vi "Menu.vi"(7 "Name (\"\" to Use UUID)":string="Menu") -> ()   [LabVIEW 2025]
doc: "Compact code template used to create a CSM module with a user interface. This template includes a user Event Structure for responding to user actions. The functionality of this template is identical to the CSM User Interface(UI) Module Template VI.\n\n\n> [!NOTE] <b>CSM Naming Rules</b>\n>\n> - CSM module name must be unique. Otherwise, CSM enters a `Critical Error` state.\n> - If the input module name is an empty string (\"\"), the system uses a UUID as the module name. Such a module is marked as standalone mode and does not appear in the module list.\n> - Worker Mode Rule: If the input module name ends with `#`, a worker mode node will be instantiated. Multiple worker mode nodes can form a worker mode module.\n> - Chain of Responsibility Mode Rule: If the input module name ends with `$` followed by a number, a chain of responsibility mode node will be instantiated. Multiple chain of responsibility mode nodes can form a chain of responsibility mode module.\n> - System-Level Module Rule: If the input module name starts with `.`, the module is a system-level module. Under default settings, such modules are not listed by the CSM - List Modules VI and are suitable for instantiating modules that run in the background.\n> - Submodule Rule: `.` is also allowed in a module name to separate the module name into multiple parts. CSM does not have strict rules for submodules. The `.` in the module name only marks the logical relationship between different modules. From an execution perspective, they are considered independent modules. The only difference is that you can obtain a list of logical submodules via the CSM - List Submodules VI.\n\n\n-- <b>Controls</b> --\n- <b>Name (\"\" to use UUID)</b>: CSM module name. Refer to <b>CSM Naming Rules</b> for module naming rules."
uses:
  <userlib>/_NEVSTOP/Communicable State Machine(CSM)/AdvanceAPI/CSM - Revert Arguments-Safe String.vi
  <userlib>/_NEVSTOP/Communicable State Machine(CSM)/_Shared/Trim Single-line Text.vi
  <userlib>/_NEVSTOP/Communicable State Machine(CSM)/AdvanceAPI/CSM - Break Down Multiple States String.vi
  <userlib>/_NEVSTOP/Communicable State Machine(CSM)/AdvanceAPI/CSM - Compact Multiple States.vi
  <userlib>/_NEVSTOP/Communicable State Machine(CSM)/AdvanceAPI/CSM - Make String Arguments Safe.vi
  <userlib>/_NEVSTOP/Communicable State Machine(CSM)/AdvanceAPI/CSM - Keywords.vi
  <userlib>/_NEVSTOP/Communicable State Machine(CSM)/Communicable State Machine.lvlib
panel:
  out "State History":string
  in  "Tab Control":enum32{"Play", "Rules"}(tab)
  in  "Rules Button":bool
  out "Records Display":string
  in  "Difficulty":enum32{"Eazy", "Hard", "Insane"}(radio)
  in  "Start Button":bool
  in  "Quit":bool
  out "Rules":string
  in  "Back Button":bool
  out "Simon Rules":string
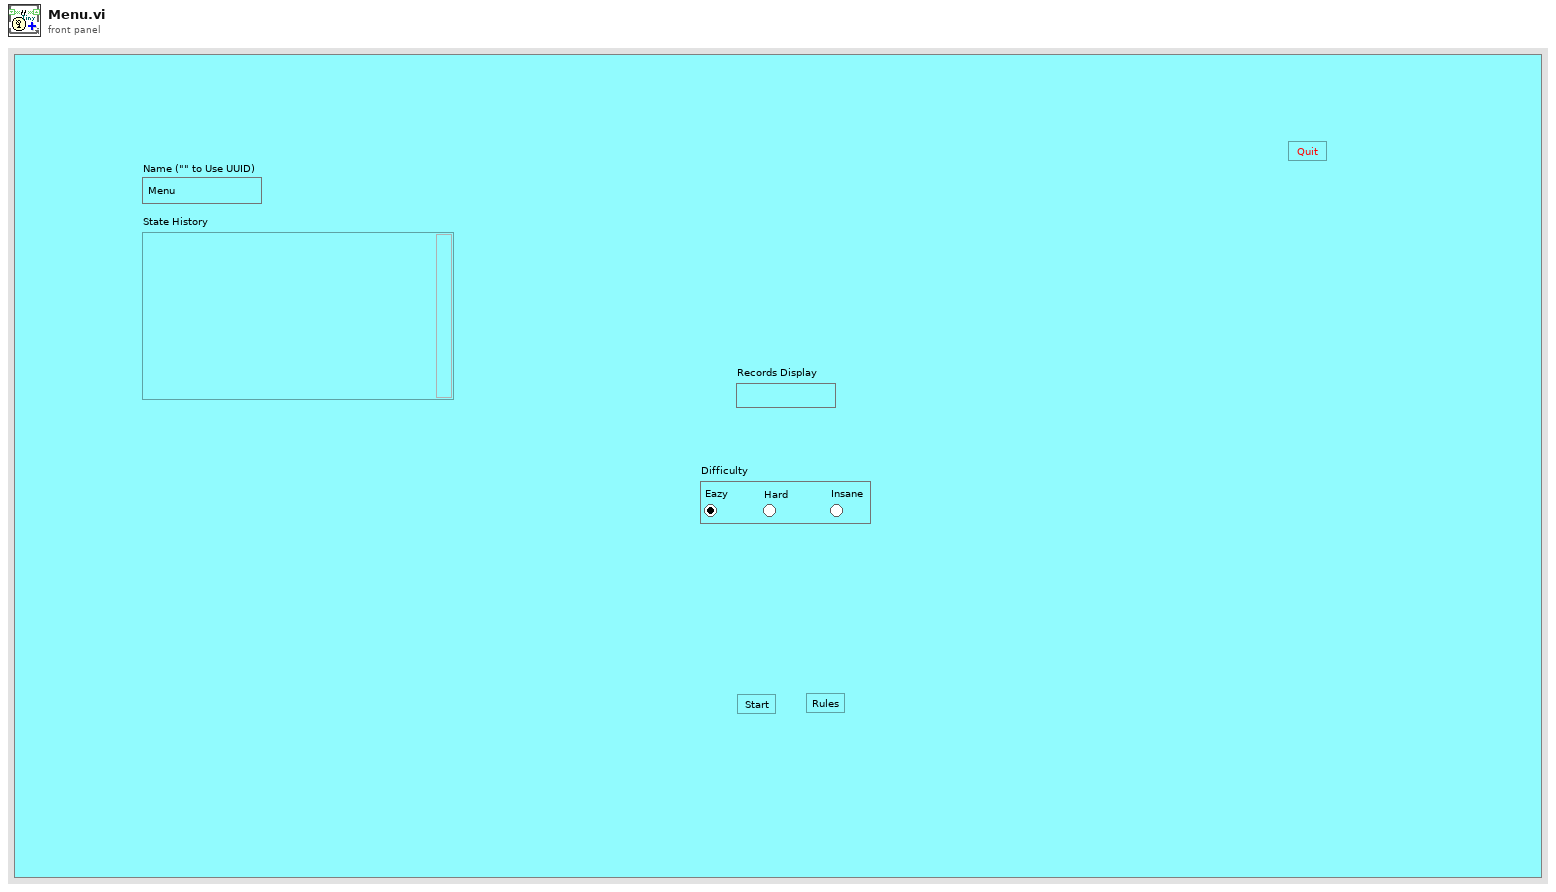
[diagram p1: front panel]
types:
  T1 = enum32{"Invalid", "Standard", "Closed", "Hidden", "Minimized", "Maximized"}
  T2 = enum32{"invalid app kind", "Development System", "Run Time System", "Student Edition", "Embedded LabVIEW", "Evaluation", "Custom"}
  T3 = typedef "Communicable State Machine.lvlib/_CSM_Response Source Message.ctl" = cluster{"‘State":string, "’Arguments":string, "’Error":errorcluster}
  T4 = cluster{"Core":cluster{"Current VI Reference":refnum<vi>, "Close Panel on Exit?":bool}, "Difficulty":i32}
  T5 = cluster{"Current VI Reference":refnum<vi>, "Close Panel on Exit?":bool}
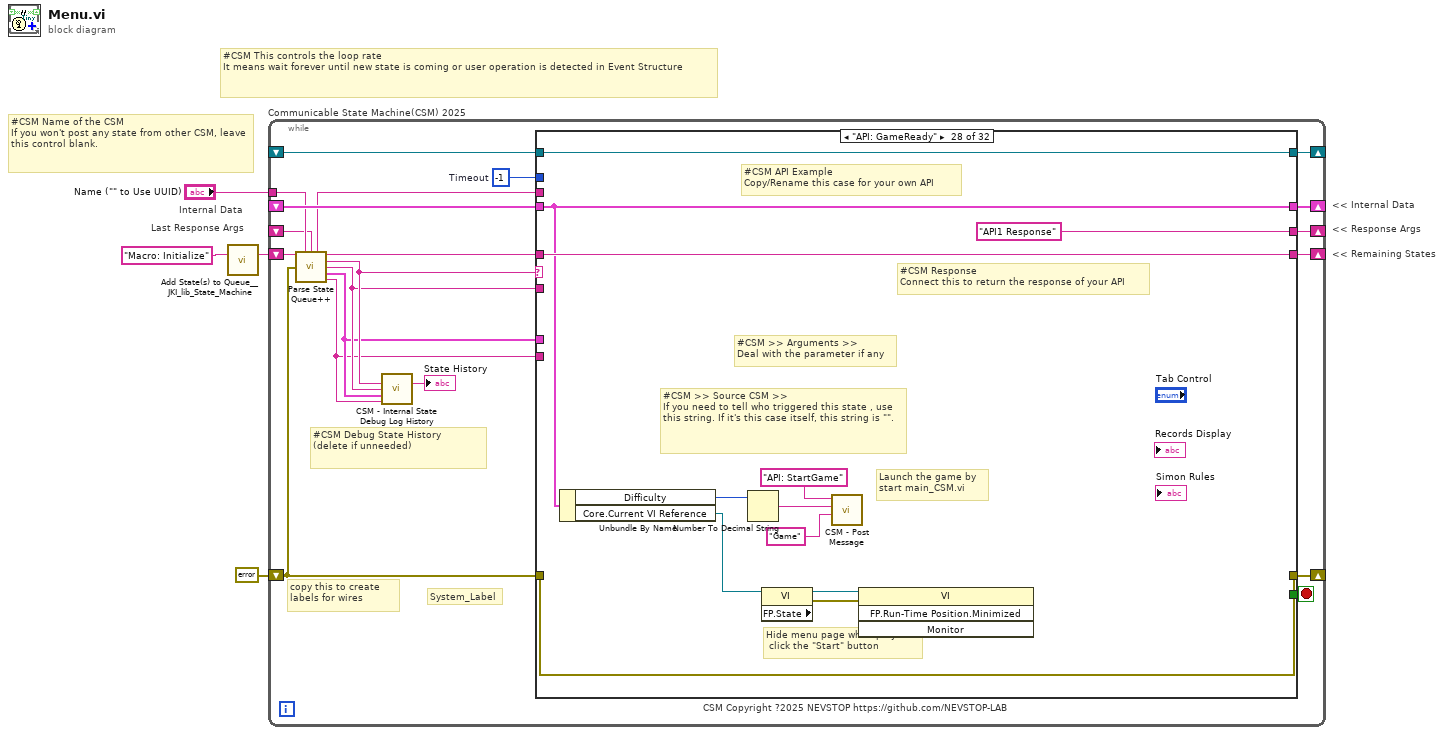
[diagram p0: block diagram]
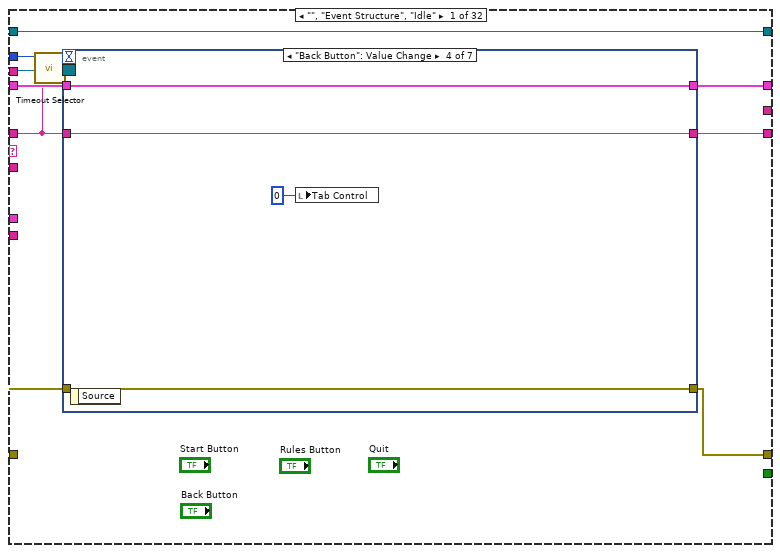
[diagram p2: hidden frame]
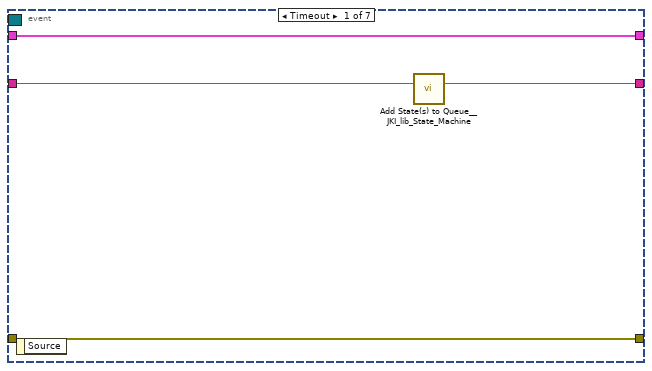
[diagram p3: hidden frame]
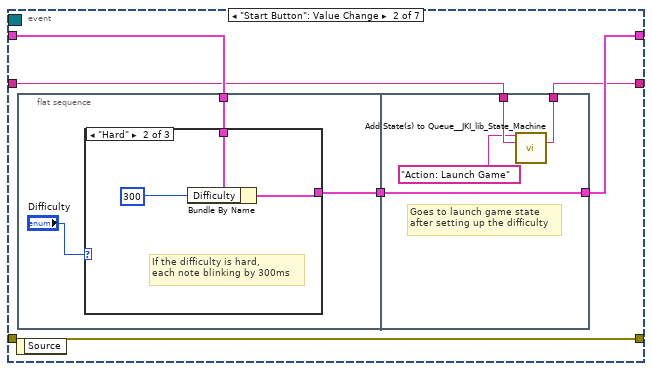
[diagram p4: hidden frame]
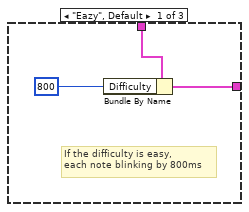
[diagram p5: hidden frame]
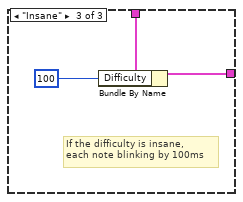
[diagram p6: hidden frame]
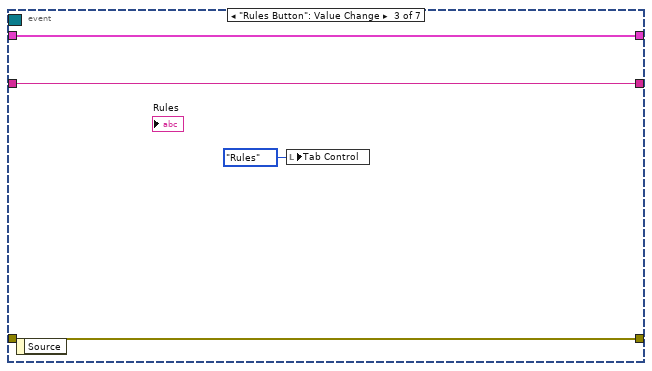
[diagram p7: hidden frame]
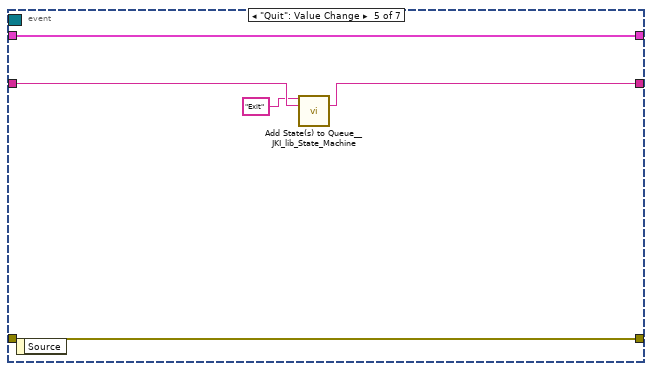
[diagram p8: hidden frame]
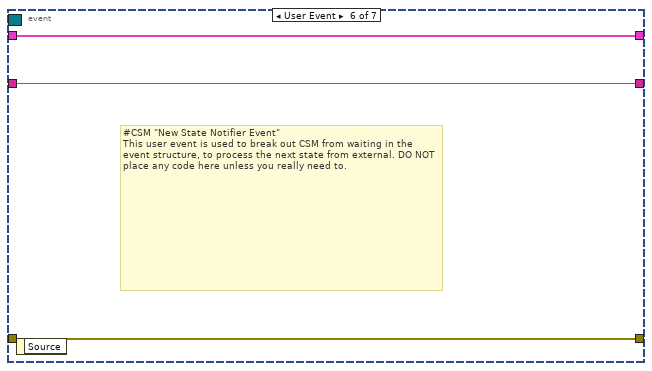
[diagram p9: hidden frame]
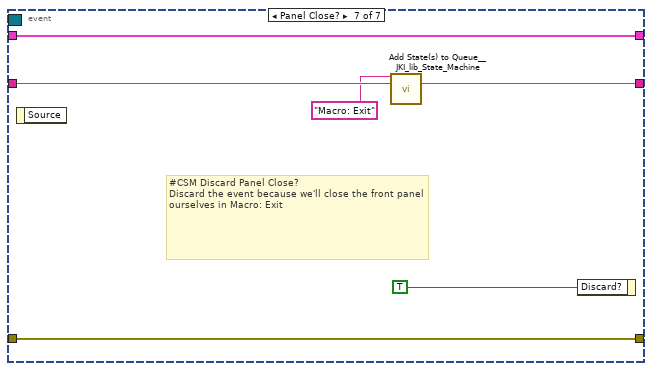
[diagram p10: hidden frame]
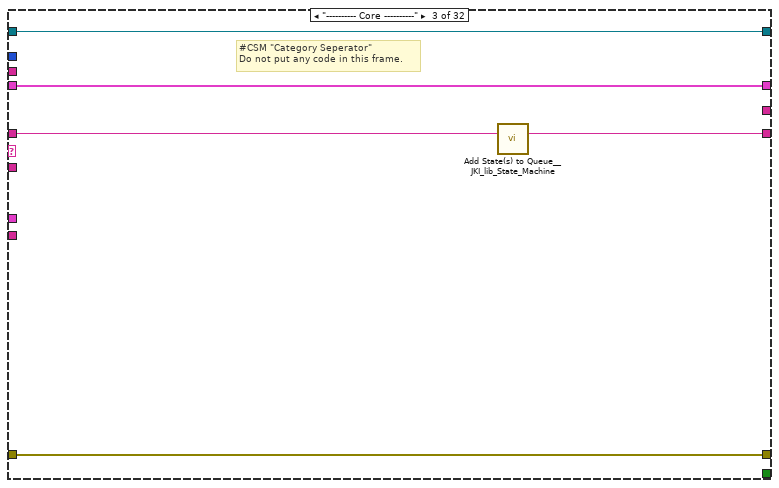
[diagram p12: hidden frame]
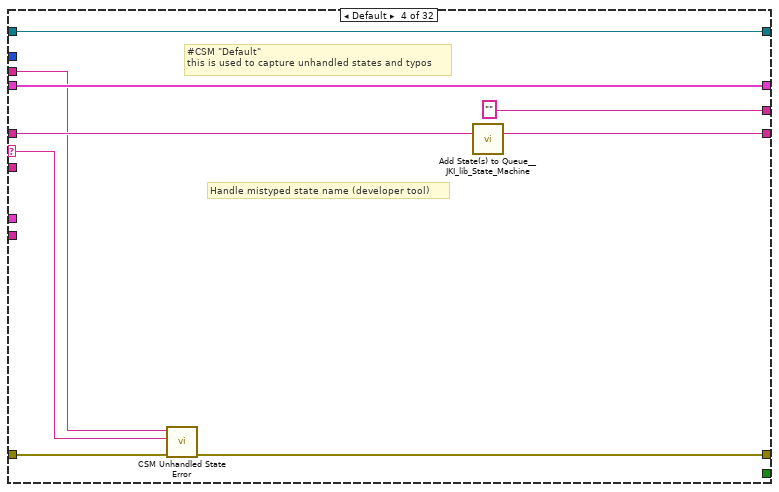
[diagram p13: hidden frame]
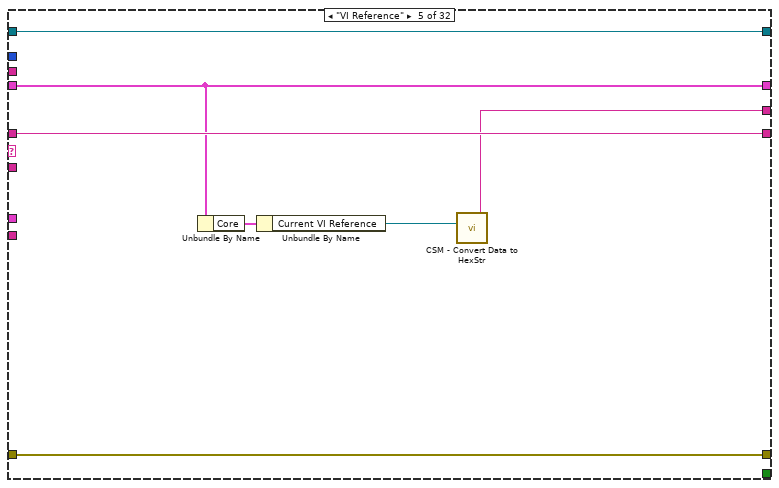
[diagram p14: hidden frame]
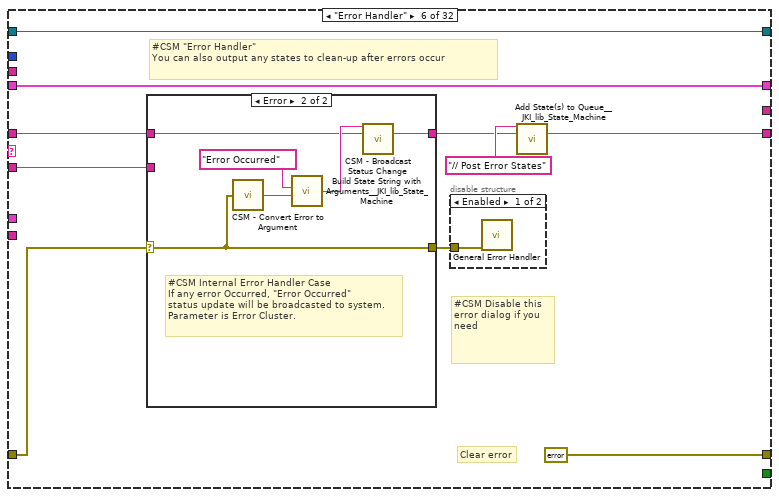
[diagram p15: hidden frame]
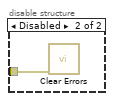
[diagram p16: hidden frame]
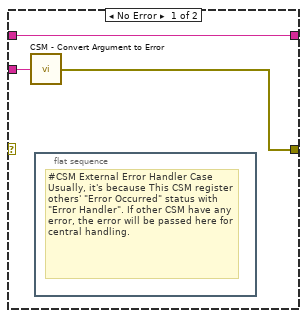
[diagram p17: hidden frame]
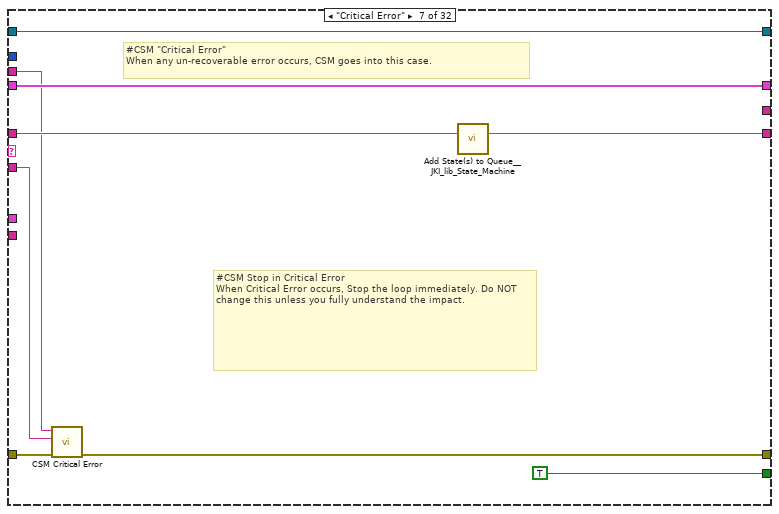
[diagram p18: hidden frame]
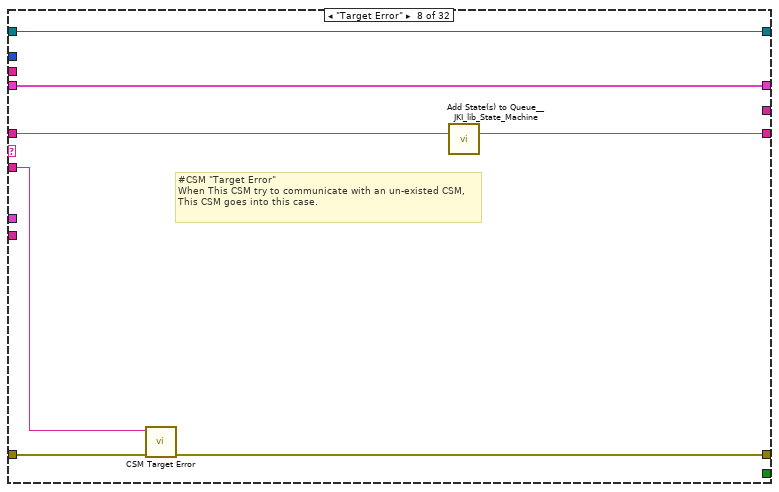
[diagram p19: hidden frame]
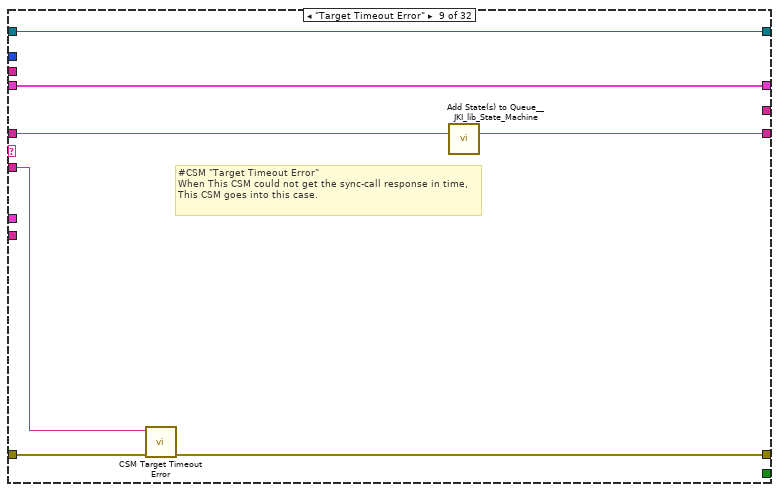
[diagram p20: hidden frame]
diagram:
  # "Last Response Args"
  # "Internal Data"
  # "#CSM Name of the CSM\nIf you won't post any state from other CSM, leave this control blank."
  # "#CSM This controls the loop rate\nIt means wait forever until new state is coming or user operation is detected in Event Structure"
  # "<< Internal Data"
  # "<< Response Args"
  # "<< Remaining States"
  n1 = call <vilib>:"Add State(s) to Queue__JKI_lib_State_Machine.vi"("State(s) in (\"\")"="Macro: Initialize" ("Init State(\"Macro: Initialize\")")) -> ("States Out"=w4:string)  [unwired: 14 in]
  n2 = while "Communicable State Machine(CSM) 2025" {
    shift-right: [w19] -> _
    shift-left: _ -> [w18]
    shift-right: [w22] -> _
    shift-left: errorcluster {"status"=FALSE, "code"=0, "source"=""} ("error out") -> [w16]
    shift-right: [w21] -> _
    shift-left: w4 -> [w23]
    tunnel: "Name (\"\" to Use UUID)" -> [w12]
    shift-right: [w15] -> _
    shift-left: _ -> [w6]
    shift-right: [w14] -> _
    shift-left: _ -> [w13]
    stop <- w20 stop-if-true
    w17 = -1  # Timeout
    # "#CSM Debug State History\n(delete if unneeded)"
    # "copy this to create labels for wires"
    # "System_Label"
    # "CSM Copyright ?2025 NEVSTOP https://github.com/NEVSTOP-LAB"
    n3 = call <userlib>:"Parse State Queue++.vi"("State Queue"=w23, "Name (\"\" to Use UUID)"=w12, "Response Arguments"=w6, "Previous Error"=w16) -> ("Name Used"=w7:string, "Remaining States"=w24:string, "Current State"=w11:string, "Arguments"=w10:string, "Additional Information"=w9:T3, "Source CSM"=w8:string)  [unwired: 6 in]
    n4 = call <userlib>:"CSM - Internal State Debug Log History.vi"("State"=w11, "Arguments (\"\")"=w10, ">> Response Source Message >>"=w9, "Source (\"\")"=w8) -> ("Debug Log"=→"State History":string)  [unwired: 11 in]
    n5 = case shown="\"API: GameReady\"" w11 {
      selector: w11 -> [_ _ _ w93 _ _ _ _ _ _ _ _ _ _ _ _ _ _ _ _ _ _ _ _ _ _ _ _ _ _ _ _]
      tunnel: w24 -> [w25 w84 w90 w98 w105 w111 w134 w140 w147 w156 w169 w184 w190 w195 w202 w209 w214 w221 w225 w231 w236 w243 w259 w329 w335 w347 w350 w362 w368 w376 w388 w393]
      tunnel: w10 -> [_ _ _ _ _ w110 w129 w139 w146 w155 _ _ _ _ _ _ _ _ _ _ _ w238 w253 _ _ _ _ _ w365 _ _ _]
      tunnel: w18 -> [w32 w83 w87 w96 w104 w115 w135 w142 w149 w158 w168 w177 w188 w192 _ w204 w211 w220 w224 w228 w234 w241 w255 w326 w332 w344 w349 w356 w367 w373 w385 w390]
      tunnel: [w31 w85 w88 w91 w106 errorcluster {"status"=FALSE, "code"=0, "source"=""} ("error out") w130 w137 w144 w161 w170 w181 w187 w193 w199 w205 w212 w215 w223 w229 w233 w239 w256 w327 w333 w345 w351 w363 w369 w374 w386 w391] -> w22
      tunnel: w16 -> [w30 w85 w88 w99 w106 w112 w136 w138 w145 _ w170 w181 w187 w193 w199 w206 w212 _ w226 w229 w233 w240 w257 w327 w333 w345 w351 w363 w369 w374 w386 w391]
      tunnel: [w33 w84 w89 w97 w105 w107 w133 w143 w150 w157 w169 w183 w189 w194 w201 w208 w213 w221 w225 w230 w235 w242 w258 w328 w334 w346 w350 w362 w368 w375 w387 w392] -> w21
      tunnel: [_ _ _ _ _ _ TRUE _ _ _ _ _ TRUE _ _ _ _ _ _ _ _ _ _ _ _ _ _ _ _ _ _ _] -> w20
      tunnel: [w29 w83 w87 w96 w104 w115 w135 w142 w149 w159 w168 w182 w188 w192 w200 w204 w211 w220 w224 w228 w234 w241 w255 w326 w332 w344 w349 w356 w367 w373 w385 w390] -> w19
      tunnel: w17 -> [w28 _ _ _ _ _ _ _ _ _ _ _ _ _ _ _ _ _ _ _ _ _ _ _ _ _ _ _ _ _ _ _]
      tunnel: w8 -> [_ _ _ _ _ _ _ _ _ w153 _ _ _ _ _ _ _ _ _ _ _ _ _ _ _ _ _ _ _ _ _ _]
      tunnel: w9 -> [_ _ _ _ _ _ _ _ _ w160 _ _ _ _ _ _ _ _ _ _ _ _ _ _ _ _ _ _ _ _ _ _]
      tunnel: [_ _ _ "" w100 _ _ _ _ _ _ _ _ _ _ _ _ _ _ _ _ _ _ _ _ _ _ "API1 Response" w364 _ _ _] -> w15
      tunnel: [w27 w82 w86 w94 w103 w114 w131 w141 w148 w162 w167 w171 w185 w191 w197 w203 w210 w219 w222 w227 w232 w237 w252 w325 w330 w337 w348 w361 w366 w372 w384 w389] -> w14
      tunnel: w13 -> [w27 w82 w86 w94 w103 w114 w131 w141 w148 w162 w167 w171 w185 w191 w197 w203 w210 _ w222 w227 w232 w237 w252 w325 w330 w337 w348 w361 w366 w372 w384 w389]
      tunnel: w7 -> [_ _ _ w92 _ _ w128 _ _ _ _ _ _ _ _ _ _ w218 _ _ _ _ _ _ _ _ _ _ _ _ _ _]
      frame "", "Event Structure", "Idle" {
        n6 = call <userlib>:"Timeout Selector.vi"("Remaining States"=w25, "Timeout Expected"=w28) -> ("Timeout"=w26:i32)  [unwired: 5 in]
        n7 = event shown="[3] \"Back Button\": Value Change" {
          selector: w27 -> [_ _ _ _ _ _ _]
          dyn-events: _ -> [_ _ _ _ _ _ _]
          timeout: w26 -> [_ _ _ _ _ _ _]
          tunnel: w25 -> [w37 w39 w63 w67 w70 w74 w81]
          tunnel: [w36 w38 w63 w67 w69 w74 w80] -> w33
          tunnel: w32 -> [w34 w42 w61 w65 w71 w75 w78]
          tunnel: [w35 w43 w62 w66 w72 w73 w79] -> w31
          tunnel: w30 -> [w35 w43 w62 w66 w72 w73 w79]
          tunnel: [w34 w41 w61 w65 w71 w75 w78] -> w29
          event Timeout {
            n8 = event-data() -> ()  [unwired: 1 in, 1 out]
            n9 = call <vilib>:"Add State(s) to Queue__JKI_lib_State_Machine.vi"("State(s) in (\"\")"=w37) -> ("States Out"=w36:string)  [unwired: 14 in]
          }
          event "Start Button": Value Change {
            n10 = event-data() -> ()  [unwired: 1 in, 1 out]
            n11 = flat-sequence {
              tunnel: w42 -> [w45]
              tunnel: [w44] -> w40
              tunnel: [w59] -> w41
              tunnel: w40 -> [w59]
              tunnel: w39 -> [w58]
              tunnel: [w57] -> w38
              frame #0 {
                n12 = case shown="\"Hard\"" "Difficulty" {
                  tunnel: w45 -> [w49 w52 w55]
                  tunnel: [w47 w51 w54] -> w44
                  frame "Eazy", Default {
                    # "If the difficulty is easy,\neach note blinking by 800ms"
                    n13 = Bundle By Name(cluster=w49, "Difficulty"=800) -> (w47:T4)
                  }
                  frame "Hard" {
                    # "If the difficulty is hard,\neach note blinking by 300ms"
                    n14 = Bundle By Name(cluster=w52, "Difficulty"=300) -> (w51:T4)
                  }
                  frame "Insane" {
                    # "If the difficulty is insane,\neach note blinking by 100ms"
                    n15 = Bundle By Name(cluster=w55, "Difficulty"=100) -> (w54:T4)
                  }
                }
              }
              frame #1 {
                # "Goes to launch game state\nafter setting up the difficulty"
                n16 = call <vilib>:"Add State(s) to Queue__JKI_lib_State_Machine.vi"("State(s) in Front (\"\")"="Action: Launch Game" ("State(s) in Front (\"\")"), "State(s) in (\"\")"=w58) -> ("States Out"=w57:string)  [unwired: 13 in]
              }
            }
          }
          event "Rules Button": Value Change {
            n17 = event-data() -> ()  [unwired: 1 in, 1 out]
            n18 = local write "Tab Control"(enum32{"Play", "Rules"}."Rules" ("Tab Control")) -> ()
          }
          event "Back Button": Value Change {
            n19 = event-data() -> ()  [unwired: 1 in, 1 out]
            n20 = local write "Tab Control"(0) -> ()
          }
          event "Quit": Value Change {
            n21 = event-data() -> ()  [unwired: 1 in, 1 out]
            n22 = call <vilib>:"Add State(s) to Queue__JKI_lib_State_Machine.vi"("State(s) in Front (\"\")"="Exit" ("State(s) in Front (\"\")"), "State(s) in (\"\")"=w70) -> ("States Out"=w69:string)  [unwired: 13 in]
          }
          event User Event {
            # "#CSM \"New State Notifier Event\"\nThis user event is used to break out CSM from waiting in the event structure, to process the next state from external. DO NOT place any code here unless you really need to."
            n23 = event-data() -> ()  [unwired: 1 in, 1 out]
          }
          event Panel Close? {
            # "#CSM Discard Panel Close?\nDiscard the event because we'll close the front panel ourselves in Macro: Exit"
            n24 = event-data() -> ()  [unwired: 1 in, 1 out]
            n25 = call <vilib>:"Add State(s) to Queue__JKI_lib_State_Machine.vi"("State(s) in Front (\"\")"="Macro: Exit", "State(s) in (\"\")"=w81) -> ("States Out"=w80:string)  [unwired: 13 in]
            n26 = event-data("Discard?"=TRUE) -> ()  [unwired: 1 in, 1 out]
          }
        }
      }
      frame "CSM Documentation" {
        # "#CSM README FIRST\n\nCommunicable State Machine(CSM) is a LabVIEW application framework that builds upon JKI State Machine(JKISM). It follows the pattern of JKISM and extends the keywords to describe message communication between modules, including concepts such as Sync-Message, Async-Message, Subscription/Unsubscription of status - essential elements for creating reusable code modules. For more information, please visit the CSM wiki: https://nevstop-lab.github.io/CSM-Wiki/\n\nFor instructions on JKI State Machine, visit: http://jki.net/state-machine/\nFor information about CSM, visit: https://github.com/NEVSTOP-LAB"
        # "#CSM \"Documentation\"\nCase for holding CSM Documenation"
      }
      frame "---------- Core ----------" {
        # "#CSM \"Category Seperator\"\nDo not put any code in this frame."
        n27 = call <vilib>:"Add State(s) to Queue__JKI_lib_State_Machine.vi"("State(s) in (\"\")"=w90) -> ("States Out"=w89:string)  [unwired: 14 in]
      }
      frame Default {
        # "#CSM \"Default\"\nthis is used to capture unhandled states and typos"
        # "Handle mistyped state name (developer tool)"
        n28 = call <userlib>:"CSM Unhandled State Error.vi"("error in (no error)"=w99, "Undefined State"=w93, "CSM Name"=w92) -> ("error out"=w91:errorcluster)  [unwired: 8 in]
        n29 = call <vilib>:"Add State(s) to Queue__JKI_lib_State_Machine.vi"("State(s) in (\"\")"=w98) -> ("States Out"=w97:string)  [unwired: 14 in]
      }
      frame "VI Reference" {
        n30 = Unbundle By Name(w104) -> ("Core"=w102:T5)
        n31 = Unbundle By Name(w102) -> ("Current VI Reference"=w101:refnum<vi>)
        n32 = call <userlib>:"CSM - Convert Data to HexStr.vi"("Variant"=w101) -> ("HEX String (0-9,A-F)"=w100:string)  [unwired: 8 in]
      }
      frame "Error Handler" {
        # "#CSM Disable this error dialog if you need"
        # "#CSM \"Error Handler\"\nYou can also output any states to clean-up after errors occur"
        # "Clear error"
        n33 = case shown="Error" w112 {
          selector: w112 -> [_ w122]
          tunnel: [w121 w124] -> w108
          tunnel: w111 -> [w121 w123]
          tunnel: w110 -> [w120 _]
          tunnel: [w119 w122] -> w113
          frame No Error {
            n34 = call <userlib>:"CSM - Convert Argument to Error.vi"("Argument"=w120) -> ("Error"=w119:errorcluster)  [unwired: 4 in]
            n35 = flat-sequence {
              frame #0 {
                # "#CSM External Error Handler Case\nUsually, it's because This CSM register others' \"Error Occurred\" status with \"Error Handler\". If other CSM have any error, the error will be passed here for central handling."
              }
            }
          }
          frame Error {
            # "#CSM Internal Error Handler Case \nIf any error Occurred, \"Error Occurred\" \nstatus update will be broadcasted to system.\nParameter is Error Cluster."
            n36 = call <userlib>:"CSM - Convert Error to Argument.vi"("Error"=w122) -> ("Argument"=w126:string)  [unwired: 4 in]
            n37 = call <vilib>:"Build State String with Arguments__JKI_lib_State_Machine.vi"("Arguments (\"\")"=w126, "State"="Error Occurred" ("Status with Arguments")) -> ("State with Arguments"=w125:string)  [unwired: 4 in]
            n38 = call <userlib>:"CSM - Broadcast Status Change.vi"("Status With Arguments"=w125, "State Queue"=w123) -> ("Remaining States"=w124:string)  [unwired: 13 in]
          }
        }
        n39 = disable-structure shown="Enabled" {
          disable-tunnel: w113 -> [w117 w118]
          frame Enabled {
            n40 = call <vilib>:"General Error Handler.vi"("error in (no error)"=w117) -> ()  [unwired: 10 in, 5 out]
          }
          frame Disabled {
            n41 = call <vilib>:"Clear Errors.vi"("error in (no error)"=w118) -> ()  [unwired: 5 in, 2 out]
          }
        }
        n42 = call <vilib>:"Add State(s) to Queue__JKI_lib_State_Machine.vi"("State(s) in Front (\"\")"="// Post Error States", "State(s) in (\"\")"=w108) -> ("States Out"=w107:string)  [unwired: 13 in]
      }
      frame "Critical Error" {
        # "#CSM Stop in Critical Error\nWhen Critical Error occurs, Stop the loop immediately. Do NOT change this unless you fully understand the impact."
        # "#CSM \"Critical Error\"\nWhen any un-recoverable error occurs, CSM goes into this case."
        n43 = call <userlib>:"CSM Critical Error.vi"("error in (no error)"=w136, "Arugments (As Reason)"=w129, "CSM Name"=w128) -> ("error out"=w130:errorcluster)  [unwired: 8 in]
        n44 = call <vilib>:"Add State(s) to Queue__JKI_lib_State_Machine.vi"("State(s) in (\"\")"=w134) -> ("States Out"=w133:string)  [unwired: 14 in]
      }
      frame "Target Error" {
        # "#CSM \"Target Error\"\nWhen This CSM try to communicate with an un-existed CSM, This CSM goes into this case."
        n45 = call <userlib>:"CSM Target Error.vi"("error in (no error)"=w138, "Arguments (As CSM Name)"=w139) -> ("error out"=w137:errorcluster)  [unwired: 9 in]
        n46 = call <vilib>:"Add State(s) to Queue__JKI_lib_State_Machine.vi"("State(s) in (\"\")"=w140) -> ("States Out"=w143:string)  [unwired: 14 in]
      }
      frame "Target Timeout Error" {
        # "#CSM \"Target Timeout Error\"\nWhen This CSM could not get the sync-call response in time, This CSM goes into this case."
        n47 = call <userlib>:"CSM Target Timeout Error.vi"("error in (no error)"=w145, "Arguments (As CSM Name)"=w146) -> ("error out"=w144:errorcluster)  [unwired: 9 in]
        n48 = call <vilib>:"Add State(s) to Queue__JKI_lib_State_Machine.vi"("State(s) in (\"\")"=w147) -> ("States Out"=w150:string)  [unwired: 14 in]
      }
      frame "Async Response", "Response" {
        n49 = Unbundle(w160) -> ("‘State"=w154:string, "’Arguments"=w152:string, "’Error"=w151:errorcluster)
        n50 = case shown="Default" w154 {
          tunnel: [w166] -> w161
          tunnel: w151 -> [w166]
          tunnel: [w165] -> w159
          tunnel: w158 -> [w165]
          tunnel: [w163] -> w157
          tunnel: w156 -> [w164]
          tunnel: w155 -> [_]
          tunnel: w153 -> [_]
          tunnel: w152 -> [_]
          frame Default {
            # "#CSM Response Comments\nAfter Message is executed, CSM goes to this state for receive the response.\n    For Async Message(->), \"Async Response\" is used. This CSM will goes to \"Async Message Posted\" immediately and receive the \"Async Response\" after the callee finishes the message.\n    For Sync Message(@),  This CSM will wait until the message is done and immediately goes to \"Response\""
            # "#CSM \"Async Response\"\nHandle Async-call Response (\"Async Response\" for ->)"
            # "#CSM \"Response\"\nHandle Sync-call Response (\"Response\" for -@)"
            n51 = call <vilib>:"Add State(s) to Queue__JKI_lib_State_Machine.vi"("State(s) in (\"\")"=w164) -> ("States Out"=w163:string)  [unwired: 14 in]
          }
        }
      }
      frame "Async Message Posted" {
        # "#CSM \"Async Message Posted\"\nAfter Async Message is posted (-> or ->| ), CSM goes to this state for post-action.\nYou can use Argument - State to tell which Async Message is called."
      }
      frame "Initialize Core Data" {
        # "#CSM \"Initialize Core Data\"\nThis is used to determine panel behavior on exit"
        # "originally closed?"
        # "exe?"
        # "If panel starts closed or is an EXE, then close it when we exit"
        n52 = property class="VI"() -> ("FP.State"=w174:T1)  [unwired: 2 in, 2 out]
        n53 = property class="App"() -> ("App.Kind"=w180:T2)  [unwired: 2 in, 2 out]
        n54 = control-ref of="Current VI Reference"() -> (w175:refnum<vi>)
        n55 = Equal?(x=w174, y=T1."Closed" ("Front Panel Window:State")) -> (x = y?=w172:bool)
        n56 = Equal?(x=w180, y=T2."Run Time System" ("Application:Kind")) -> (x = y?=w178:bool)
        n57 = Or(x=w172, y=w178) -> (x .or. y?=w176:bool)
        n58 = Bundle By Name(cluster=w177, "Core.Current VI Reference"=w175, "Core.Close Panel on Exit?"=w176) -> (w182:T4)
        n59 = call <vilib>:"Add State(s) to Queue__JKI_lib_State_Machine.vi"("State(s) in (\"\")"=w184) -> ("States Out"=w183:string)  [unwired: 14 in]
      }
      frame "Exit" {
        # "#CSM \"Exit\"\nCase for exiting the loop. No errors that occur here will be handled."
        n60 = call <vilib>:"Add State(s) to Queue__JKI_lib_State_Machine.vi"("State(s) in (\"\")"=w190) -> ("States Out"=w189:string)  [unwired: 14 in]
      }
      frame "---------- Data ----------" {
        # "#CSM \"Category Seperator\"\nDo not put any code in this frame."
        n61 = call <vilib>:"Add State(s) to Queue__JKI_lib_State_Machine.vi"("State(s) in (\"\")"=w195) -> ("States Out"=w194:string)  [unwired: 14 in]
      }
      frame "Data: Initialize" {
        w196 = 500  # Difficulty
        w198 = T5 {"Current VI Reference"=refnum, "Close Panel on Exit?"=FALSE}  # Core
        # "#CSM do not delete - used by framework"
        # "#CSM Expand Bundle to add new data elements to shift register data."
        # "#CSM Add new data here."
        # "Initialize the shift-register data, here.\n(data names are defined by what you wire into the bundle function)"
        n62 = Bundle("Core"=w198, "Difficulty"=w196) -> (w200:T4)  [unwired: 1 in]
        n63 = call <vilib>:"Add State(s) to Queue__JKI_lib_State_Machine.vi"("State(s) in (\"\")"=w202) -> ("States Out"=w201:string)  [unwired: 14 in]
      }
      frame "Data: Cleanup" {
        # "Cleanup any data and references, here.\n(this is called automatically, by the Macro: Exit)"
        n64 = Unbundle By Name(w204) -> ("Core.Current VI Reference"=w207:refnum<vi>)
        n65 = Close Reference(reference=w207, error in (no error)=w206) -> (error out=w205:errorcluster)
        n66 = call <vilib>:"Add State(s) to Queue__JKI_lib_State_Machine.vi"("State(s) in (\"\")"=w209) -> ("States Out"=w208:string)  [unwired: 14 in]
      }
      frame "---------- Events ----------" {
        # "#CSM \"Category Seperator\"\nDo not put any code in this frame."
        n67 = call <vilib>:"Add State(s) to Queue__JKI_lib_State_Machine.vi"("State(s) in (\"\")"=w214) -> ("States Out"=w213:string)  [unwired: 14 in]
      }
      frame "Events: Register" {
        # "#CSM \"Events: Register\"\nRegister user event. New Message Event is registered to break CSM waiting in event structure by default."
        # "#CSM Register New Message Event\nRegister message event to break Waiting in Event structure."
        n68 = call <userlib>:"CSM - Get New State Notifier Event.vi"("Name (\"\" to Use UUID)"=w218) -> ("error out"=w216:errorcluster, "New State Notifier Event"=w217:refnum<user-event>)  [unwired: 9 in]
        n69 = register-events(error in=w216, w217) -> (reference out=w219:refnum<event-registration>, error out=w215:errorcluster)  [unwired: 1 in]
      }
      frame "Events: Unregister" {
        # "#CSM \"Events: Unregister\"\nUnregister user event."
        n70 = Unregister For Events(event registration refnum=w222, error in=w226) -> (error out=w223:errorcluster)
      }
      frame "---------- UI ----------" {
        # "#CSM \"Category Seperator\"\nDo not put any code in this frame."
        n71 = call <vilib>:"Add State(s) to Queue__JKI_lib_State_Machine.vi"("State(s) in (\"\")"=w231) -> ("States Out"=w230:string)  [unwired: 14 in]
      }
      frame "UI: Initialize" {
        # "#CSM \"UI: Initialize\"\nInitialize the User Interface, here.\n(this is called automatically, by the Macro: Init)"
        n72 = call <vilib>:"Add State(s) to Queue__JKI_lib_State_Machine.vi"("State(s) in (\"\")"=w236) -> ("States Out"=w235:string)  [unwired: 14 in]
      }
      frame "UI: Cursor Set" {
        # "#CSM \"UI: Cursor Set\"\nSet and Unset Cursor Busy.\n(Usage: \"UI: Cursor Set >> Busy|Idle\")"
        # "Argument"
        n73 = disable-structure shown="Default" {
          disable-tunnel: w240 -> [w246 w251]
          disable-tunnel: [w245 w251] -> w239
          disable-tunnel: w238 -> [w244 _]
          frame condition #0 (active) {
            n74 = case shown="\"Idle\", Default" w244 {
              tunnel: w246 -> [w248 w250]
              tunnel: [w247 w249] -> w245
              frame "Idle", Default {
                n75 = call <vilib>:"Unset Busy.vi"("error in (no error)"=w248) -> ("error out"=w247:errorcluster)  [unwired: 10 in]
              }
              frame "Busy" {
                n76 = call <vilib>:"Set Busy.vi"("error in (no error)"=w250) -> ("error out"=w249:errorcluster)  [unwired: 9 in, 1 out]
              }
            }
          }
          frame condition #1 {
          }
        }
        n77 = call <vilib>:"Add State(s) to Queue__JKI_lib_State_Machine.vi"("State(s) in (\"\")"=w243) -> ("States Out"=w242:string)  [unwired: 14 in]
      }
      frame "UI: Front Panel State" {
        # "#CSM \"UI: Front Panel State\"\nSet Front Panel Open or Closed\n(Usage: \"UI: Front Panel State >> Open|Close\")"
        # "Argument"
        n78 = Unbundle By Name(w255) -> ("Core.Current VI Reference"=w254:refnum<vi>)
        n79 = call <vilib>:"Add State(s) to Queue__JKI_lib_State_Machine.vi"("State(s) in (\"\")"=w259) -> ("States Out"=w258:string)  [unwired: 14 in]
        n80 = case shown="\"Open\", \"Standard\", Default" w253 {
          tunnel: w257 -> [w265 w280 w291 w304 w317]
          tunnel: [w267 w281 w293 w306 w319] -> w256
          tunnel: w254 -> [w266 w278 w292 w305 w318]
          frame "Open", "Standard", Default {
            w260 = T1."Maximized" ("State")
            n81 = property class="VI"(reference=w266, error in=w265) -> (reference out=w263:refnum<vi>, error out=w264:errorcluster, "FP.State"=w262:T1)
            n82 = Not Equal?(x=w262, y=w260) -> (x != y?=w261:bool)
            n83 = case shown="True" w261 {
              tunnel: [w271 w273] -> w267
              tunnel: w264 -> [w270 w273]
              tunnel: w263 -> [w269 _]
              tunnel: w260 -> [w268 _]
              frame True {
                (unwired) TRUE
                n84 = invoke class="VI" method="FP.Open"(reference=w269, error in=w270, "Activate"=TRUE, "State"=w268) -> (error out=w271:errorcluster)  [unwired: 1 in, 4 out]
              }
              frame False {
              }
            }
          }
          frame "Close", "Closed" {
            n85 = property class="VI"(reference=w278, error in=w280) -> (reference out=w277:refnum<vi>, error out=w279:errorcluster, "FP.State"=w275:T1)
            n86 = Not Equal?(x=w275, y=T1."Closed" ("Front Panel Window:State")) -> (x != y?=w274:bool)
            n87 = case shown="False" w274 {
              tunnel: [w282 w285] -> w281
              tunnel: w279 -> [w282 w284]
              tunnel: w277 -> [_ w283]
              frame False {
              }
              frame True {
                n88 = invoke class="VI" method="FP.Close"(reference=w283, error in=w284) -> (error out=w285:errorcluster)  [unwired: 1 in, 2 out]
              }
            }
          }
          frame "Hidden", "Hide" {
            w286 = T1."Hidden" ("State")
            n89 = property class="VI"(reference=w292, error in=w291) -> (reference out=w289:refnum<vi>, error out=w290:errorcluster, "FP.State"=w288:T1)
            n90 = Not Equal?(x=w288, y=w286) -> (x != y?=w287:bool)
            n91 = case shown="True" w287 {
              tunnel: [w297 w298] -> w293
              tunnel: w290 -> [w296 w298]
              tunnel: w289 -> [w295 _]
              tunnel: w286 -> [w294 _]
              frame True {
                n92 = invoke class="VI" method="FP.Open"(reference=w295, error in=w296, "State"=w294) -> (error out=w297:errorcluster)  [unwired: 2 in, 4 out]
              }
              frame False {
              }
            }
          }
          frame "Minimize", "Minimized" {
            w299 = T1."Minimized" ("State")
            n93 = property class="VI"(reference=w305, error in=w304) -> (reference out=w302:refnum<vi>, error out=w303:errorcluster, "FP.State"=w301:T1)
            n94 = Not Equal?(x=w301, y=w299) -> (x != y?=w300:bool)
            n95 = case shown="True" w300 {
              tunnel: [w310 w311] -> w306
              tunnel: w303 -> [w309 w311]
              tunnel: w302 -> [w308 _]
              tunnel: w299 -> [w307 _]
              frame True {
                n96 = invoke class="VI" method="FP.Open"(reference=w308, error in=w309, "State"=w307) -> (error out=w310:errorcluster)  [unwired: 2 in, 4 out]
              }
              frame False {
              }
            }
          }
          frame "Maximize", "Maximized" {
            w312 = T1."Maximized" ("State")
            n97 = property class="VI"(reference=w318, error in=w317) -> (reference out=w315:refnum<vi>, error out=w316:errorcluster, "FP.State"=w314:T1)
            n98 = Not Equal?(x=w314, y=w312) -> (x != y?=w313:bool)
            n99 = case shown="True" w313 {
              tunnel: [w323 w324] -> w319
              tunnel: w316 -> [w322 w324]
              tunnel: w315 -> [w321 _]
              tunnel: w312 -> [w320 _]
              frame True {
                n100 = invoke class="VI" method="FP.Open"(reference=w321, error in=w322, "State"=w320) -> (error out=w323:errorcluster)  [unwired: 2 in, 4 out]
              }
              frame False {
              }
            }
          }
        }
      }
      frame "---------- Macro ----------" {
        # "#CSM \"Category Seperator\"\nDo not put any code in this frame."
        n101 = call <vilib>:"Add State(s) to Queue__JKI_lib_State_Machine.vi"("State(s) in (\"\")"=w329) -> ("States Out"=w328:string)  [unwired: 14 in]
      }
      frame "Macro: Initialize" {
        w331 = "Data: Initialize\nInitialize Core Data\nEvents: Register\nUI: Initialize\nUI: Front Panel State >> Open"  # Data: Initialize Initialize Core Data Events: Register UI: Initialize UI: Front Panel State >> Open
        # "#CSM \"Macro: Initialize\"\nInitialization Macro (This is called once, when the VI starts)"
        n102 = call <vilib>:"Add State(s) to Queue__JKI_lib_State_Machine.vi"("State(s) in Front (\"\")"=w331, "State(s) in (\"\")"=w335) -> ("States Out"=w334:string)  [unwired: 13 in]
      }
      frame "Macro: Exit" {
        # "#CSM \"Macro: Exit\"\nExit Macro (This is called once, when the VI exits)"
        n103 = Unbundle By Name(w344) -> ("Core.Close Panel on Exit?"=w343:bool)
        n104 = Select(t="UI: Front Panel State >> Close", s=w343, f="") -> (s? t:f=w340:string)
        n105 = call <vilib>:"Add State(s) to Queue__JKI_lib_State_Machine.vi"("State(s) in Front (\"\")"="//Exit Sub-Modules ", "State(s) in (\"\")"=w340, "State(s) at Back (\"\")"="Data: Cleanup\nEvents: Unregister\nExit") -> ("States Out"=w338:string)  [unwired: 12 in]
        n106 = call <vilib>:"Add State(s) to Queue__JKI_lib_State_Machine.vi"("State(s) in Front (\"\")"=w338, "State(s) in (\"\")"=w347) -> ("States Out"=w346:string)  [unwired: 13 in]
      }
      frame "---------- API ----------" {
        # "#CSM \"Category Seperator\"\nDo not put any code in this frame."
      }
      frame "API: GameReady" {
        # "Launch the game by\nstart main_CSM.vi"
        # "Hide menu page when player\n click the \"Start\" button"
        # "#CSM API Example\nCopy/Rename this case for your own API"
        # "#CSM Response\nConnect this to return the response of your API"
        # "#CSM >> Source CSM >>\nIf you need to tell who triggered this state , use this string. If it's this case itself, this string is \"\"."
        # "#CSM >> Arguments >>\nDeal with the parameter if any"
        n107 = Unbundle By Name(w356) -> ("Difficulty"=w355:i32, "Core.Current VI Reference"=w354:refnum<vi>)
        n108 = Number To Decimal String(number=w355) -> (decimal integer string=w359:string)  [unwired: 1 in]
        n109 = property class="VI" props=["FP.State"](reference=w354) -> (reference out=w353:refnum<vi>, error out=w352:errorcluster)  [unwired: 1 in, 1 out]
        n110 = call <userlib>:"CSM - Post Message.vi"("Target Module"="Game", "Arguments (\"\")"=w359, "State"="API: StartGame") -> ()  [unwired: 8 in, 1 out]
        n111 = invoke class="VI" method="FP.Run-Time Position.Minimized"(reference=w353, error in=w352) -> ()  [unwired: 2 in, 4 out]
      }
      frame "API: API2" {
        # "#CSM API Example\nCopy/Rename this case for your own API"
        # "unpack Hex String  to Variant\nif complex parameter is needed."
        n112 = call <userlib>:"CSM - Convert HexStr to Data.vi"("HEX String"=w365) -> ()  [unwired: 7 in, 2 out]
        n113 = disable-structure shown="Disabled" {
          disable-tunnel: [w370 "API2 Response"] -> w364
          frame Disabled {
            # "pack variant to hexstr \nif complex response is needed."
            # "complex Response"
            n114 = call <userlib>:"CSM - Convert Data to HexStr.vi"() -> ("HEX String (0-9,A-F)"=w370:string)  [unwired: 9 in]
          }
          frame Enabled {
          }
        }
      }
      frame "---------- Action ----------" {
        # "#CSM \"Category Seperator\"\nDo not put any code in this frame."
        n115 = call <vilib>:"Add State(s) to Queue__JKI_lib_State_Machine.vi"("State(s) in (\"\")"=w376) -> ("States Out"=w375:string)  [unwired: 14 in]
      }
      frame "Action: Launch Game" {
        # "#CSM \"Internal State\"\nThis category is used for holding internal states"
        n116 = call <vilib>:"Application Directory.vi"() -> ("Application Directory"=w379:path)
        n117 = Build Path(base path=w379, name or relative path=path "main_CSM.vi") -> (appended path=w377:path)
        n118 = Open VI Reference(vi path=w377) -> (vi reference=w383:refnum<vi>, error out=w380:errorcluster)  [unwired: 5 in]
        n119 = invoke class="VI" method="Run VI"(reference=w383, error in=w380, "Wait until done"=FALSE, "Auto Dispose Ref"=TRUE) -> ()  [unwired: 1 in, 5 out]
        n120 = call <vilib>:"Add State(s) to Queue__JKI_lib_State_Machine.vi"("State(s) in (\"\")"=w388) -> ("States Out"=w387:string)  [unwired: 14 in]
      }
      frame "Action: action2" {
        # "#CSM \"Internal State\"\nThis category is used for holding internal states"
        n121 = call <vilib>:"Add State(s) to Queue__JKI_lib_State_Machine.vi"("State(s) in (\"\")"=w393) -> ("States Out"=w392:string)  [unwired: 14 in]
      }
    }
  }
